vi "Run_Load_SampleImages.vi"(8 "error in (no error)":errorcluster caption="entrée d'erreur (pas d'erreur)", 11 "Load_SampleImages.lvclass":refnum<class "Load_SampleImages.lvclass">) -> (0 "error out":errorcluster caption="sortie d'erreur", 3 "Load_SampleImages.lvclass":refnum<class "Load_SampleImages.lvclass">)   [LabVIEW 2020, in "Load_SampleImages.lvclass"]
uses:
  Load_SampleImages.lvclass
  Load_SampleImages.lvclass/Load_SampleImages.ctl
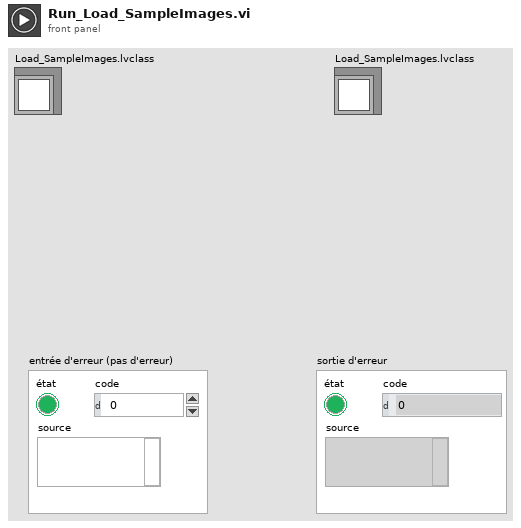
[diagram p1: front panel]
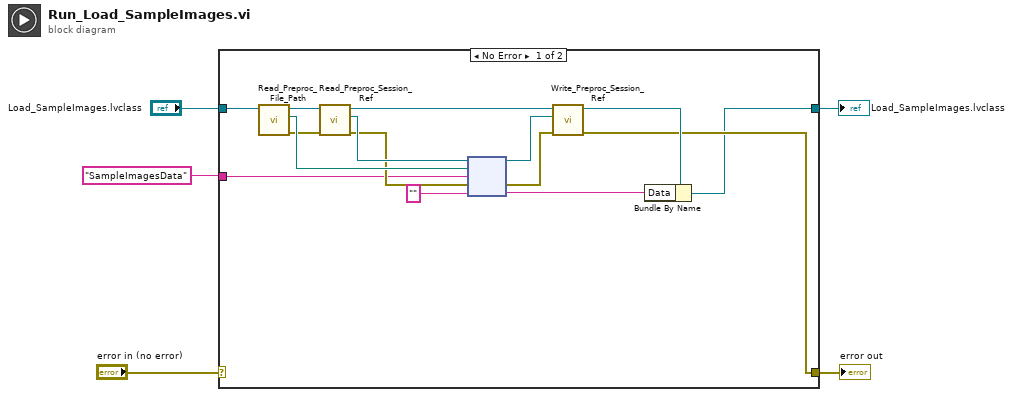
[diagram p0: block diagram]
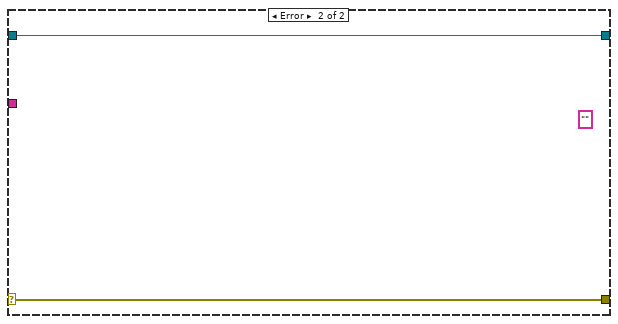
[diagram p2: hidden frame]
diagram:
  n1 = case shown="No Error" "error in (no error)" {
    selector: "error in (no error)" -> [_ w22]
    tunnel: [w8 w22] -> w4
    tunnel: [w6 w21] -> w2
    tunnel: "Load_SampleImages.lvclass" -> [w9 w21]
    tunnel: "SampleImagesData" -> [w10 _]
    frame No Error {
      n2 = call-dynamic "Read_Preproc_File_Path.vi"("Python in"=w9) -> ("error out"=w15:errorcluster, "File_Path"=w18:path, "Python out"=w20:refnum<class "Load_SampleImages.lvclass">)  [unwired: 8 in]
      n3 = call-dynamic "Read_Preproc_Session_Ref.vi"("error in (no error)"=w15, "Python in"=w20) -> ("error out"=w16:errorcluster, "Session_ref"=w17:refnum<k35>, "Python out"=w19:refnum<class "Load_SampleImages.lvclass">)  [unwired: 7 in]
      n4 = node(w17, w18, w10, w16, "") -> (w12:refnum<k35>, w14:errorcluster, w7:string)  [unwired: 2 out]
      n5 = call-dynamic "Write_Preproc_Session_Ref.vi"("error in (no error)"=w14, "Session_ref"=w12, "Python in"=w19) -> ("error out"=w8:errorcluster, "Python out"=w11:refnum<class "Load_SampleImages.lvclass">)  [unwired: 7 in]
      n6 = Bundle By Name(cluster=w11, "Data"=w7) -> (w6:refnum<class "Load_SampleImages.lvclass">)
    }
    frame Error {
      (unwired) ""
    }
  }
  "error out" <- w4
  "Load_SampleImages.lvclass" <- w2
